vi "Measurement Logic.vi"(8 "error in":errorcluster, 10 "Measurement Context":refnum<class "MeasurementContext.lvclass">, 11 "Measurement Configuration":T2={"pin_name"="Pin1", "measurement_type"=1, "range"=10.0, "resolution_digits"=5.5} {"measurement_type" items=["DC Volts"=1, "AC Volts"=2, "DC Current"=3, "AC Current"=4, "2-Wire Resistance"=5, "4-Wire Resistance"=101, "Frequency"=104, "Period"=105, "AC Volts DC Coupled"=1001, "Diode"=1002, "Waveform Voltage"=1003, "Waveform Current"=1004, "Capacitance"=1005, "Inductance"=1006, "Temperature"=108]}) -> (0 "error out":errorcluster, 2 "Measurement Context out":refnum<class "MeasurementContext.lvclass">, 3 "Measurement Results":T1)   [LabVIEW 2020, in "NI-DMM Measurement.lvlib"]
uses:
  NI-DMM Measurement.lvlib
  Measurement Configuration.ctl
  Measurement Results.ctl
  RPC Service/MeasurementContext/MeasurementContext.lvclass
  measurement-services-labview-DCPowerExample/Source/Session Management Client_lv/MeasurementLink Session Management Client/RPC Messages/ni_measurementlink_sessionmanagement_v1_ReserveSessionsRequest.ctl
  measurement-services-labview-DCPowerExample/Source/Session Management Client_lv/MeasurementLink Session Management Client/RPC Messages/ni_measurementlink_PinMapContext.ctl
  <vilib>/MeasurementLink/Discovery Client/RPC Messages/ni_measurementlink_discovery_v1_ResolveServiceRequest.ctl
  measurement-services-labview-DCPowerExample/Source/Session Management Client_lv/MeasurementLink Session Management Client/MeasurementLink Session Management Client.lvlib
  <vilib>/MeasurementLink/Discovery Client/MeasurementLink Discovery Client.lvlib
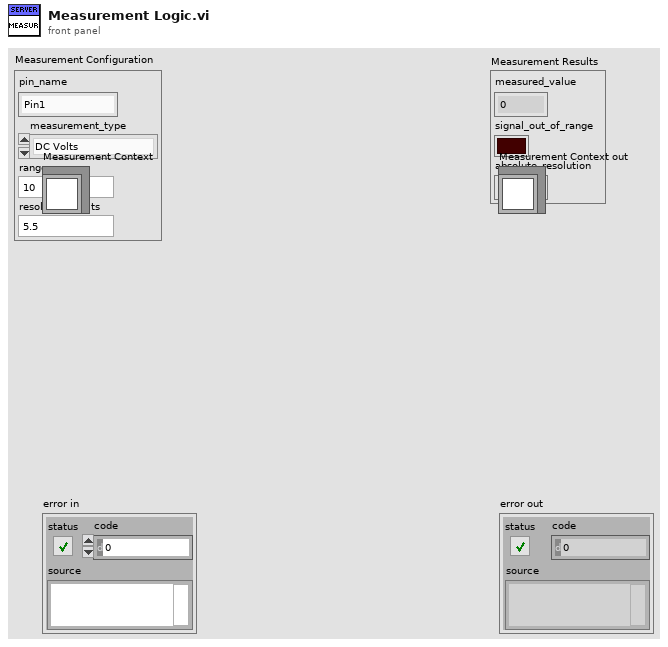
[diagram p1: front panel]
types:
  T1 = typedef "NI-DMM Measurement.lvlib/Measurement Results.ctl" = cluster{"measured_value":dbl, "signal_out_of_range":bool, "absolute_resolution":dbl}
  T2 = typedef "NI-DMM Measurement.lvlib/Measurement Configuration.ctl" = cluster{"pin_name":string, "measurement_type":i32, "range":dbl, "resolution_digits":dbl}
  T3 = typedef "MeasurementLink Discovery Client.lvlib/ni_measurementlink_discovery_v1_ResolveServiceRequest.ctl" = cluster{"provided_interface":string, "service_class":string}
  T4 = typedef "MeasurementLink Session Management Client.lvlib/ni_measurementlink_sessionmanagement_v1_ReserveSessionsRequest.ctl" = cluster{"pin_map_context":T5, "pin_or_relay_names":string[], "instrument_type_id":string, "timeout_in_milliseconds":i32}
  T5 = typedef "MeasurementLink Session Management Client.lvlib/ni_measurementlink_PinMapContext.ctl" = cluster{"pin_map_id":string, "sites":i32[]}
  T6 = typedef "MeasurementLink Measurement Server Internal.lvlib/ni_measurementlink_PinMapContext.ctl" = cluster{"pin_map_id":string, "sites":i32[]}
  T7 = typedef "grpc-lvsupport-release.lvlib/grpcId.ctl" = u64
  T8 = typedef "MeasurementLink Discovery Client.lvlib/ni_measurementlink_discovery_v1_ServiceLocation.ctl" = cluster{"location":string, "insecure_port":string, "ssl_authenticated_port":string}
  T9 = typedef "MeasurementLink Session Management Client.lvlib/ni_measurementlink_sessionmanagement_v1_ReserveSessionsResponse.ctl" = cluster{"sessions":T10[]}
  T10 = typedef "MeasurementLink Session Management Client.lvlib/ni_measurementlink_sessionmanagement_v1_SessionInformation.ctl" = cluster{"session":T11, "resource_name":string, "channel_list":string, "instrument_type_id":string, "session_exists":bool}
  T11 = typedef "MeasurementLink Session Management Client.lvlib/ni_measurementlink_sessionmanagement_v1_Session.ctl" = cluster{"name":string}
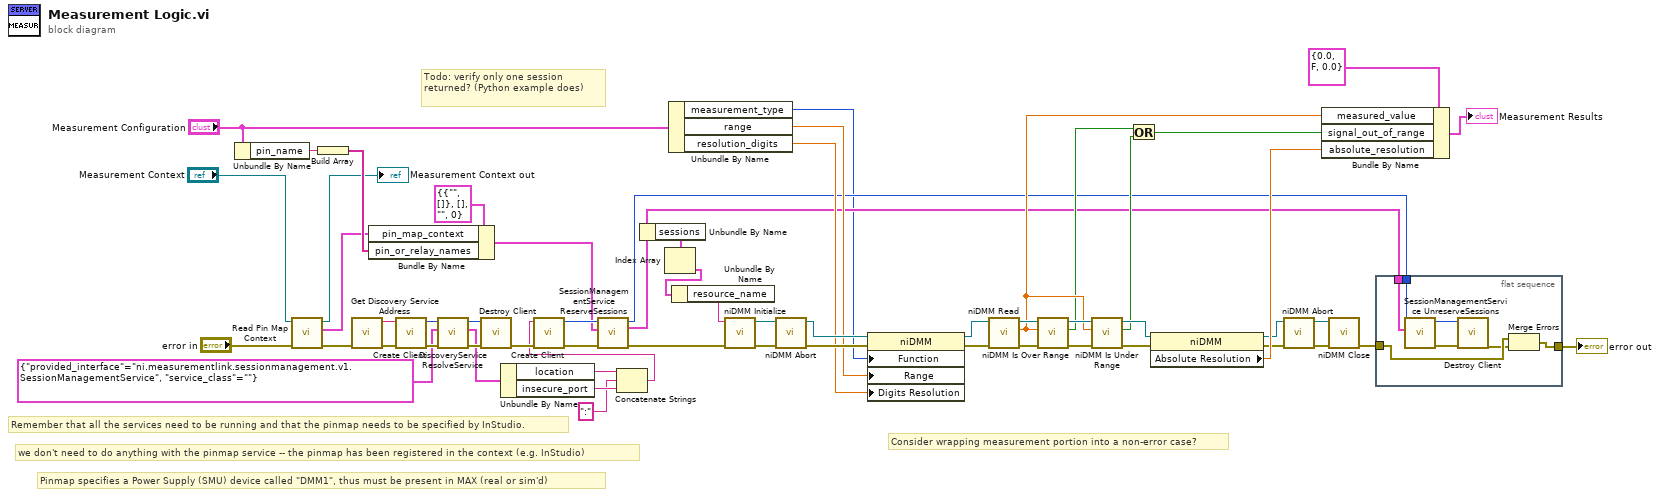
[diagram p0: block diagram]
diagram:
  # "Consider wrapping measurement portion into a non-error case?"
  # "Todo: verify only one session returned? (Python example does)"
  # "Pinmap specifies a Power Supply (SMU) device called \"DMM1\", thus must be present in MAX (real or sim'd)"
  # "Remember that all the services need to be running and that the pinmap needs to be specified by InStudio."
  # "we don't need to do anything with the pinmap service -- the pinmap has been registered in the context (e.g. InStudio)"
  n1 = Unbundle By Name("Measurement Configuration") -> ("pin_name"=w59:string)
  n2 = call-dynamic "Read Pin Map Context.vi"("error in (no error)"="error in", "MeasurementContext in"="Measurement Context") -> ("error out"=w37:errorcluster, "pin map context"=w54:T6, "MeasurementContext out"=→"Measurement Context out":refnum<class "MeasurementContext.lvclass">)  [unwired: 7 in]
  n3 = Build Array(w59) -> (w58:string[])
  n4 = call "Get Discovery Service Address.vi"("error in"=w37) -> ("error out"=w36:errorcluster, "address"=w35:string)  [unwired: 9 in]
  n5 = Bundle By Name(cluster=T4 {"pin_map_context"={"pin_map_id"="", "sites"=[]}, "pin_or_relay_names"=[], "instrument_type_id"="", "timeout_in_milliseconds"=0} ("Request Data"), "pin_map_context"=w54, "pin_or_relay_names"=w58) -> (w50:T4)
  n6 = call <vilib>:"Create Client.vi"("error in"=w36, "address"=w35) -> ("error out"=w47:errorcluster, "gRPC ID Out"=w46:T7)  [unwired: 8 in]
  n7 = call <vilib>:"DiscoveryService ResolveService.vi"("error in"=w47, "Request Data"=T3 {"provided_interface"="ni.measurementlink.sessionmanagement.v1.SessionManagementService", "service_class"=""}, "gRPC ID"=w46) -> ("error out"=w44:errorcluster, "Response Data"=w39:T8, "gRPC ID out"=w45:T7)  [unwired: 6 in]
  n8 = call <vilib>:"Destroy Client.vi"("error in"=w44, "gRPC ID"=w45) -> ("error out"=w43:errorcluster)  [unwired: 9 in]
  n9 = Unbundle By Name(w39) -> ("location"=w42:string, "insecure_port"=w41:string)
  n10 = Concatenate Strings(w42, ":" ("string"), w41) -> (w38:string)
  n11 = call <vilib>:"Create Client.vi"("error in"=w43, "address"=w38) -> ("error out"=w56:errorcluster, "gRPC ID Out"=w57:T7)  [unwired: 8 in]
  n12 = call "SessionManagementService ReserveSessions.vi"("error in"=w56, "Request Data"=w50, "gRPC ID"=w57) -> ("error out"=w31:errorcluster, "Response Data"=w4:T9, "gRPC ID out"=w7:T7)  [unwired: 6 in]
  n13 = Unbundle By Name(w4) -> ("sessions"=w49:T10[])
  n14 = Index Array(array=w49) -> (element=w48:T10)  [unwired: 1 in]
  n15 = Unbundle By Name("Measurement Configuration") -> ("measurement_type"=w3:i32, "range"=w24:dbl, "resolution_digits"=w23:dbl)
  n16 = Unbundle By Name(w48) -> ("resource_name"=w30:string)
  n17 = call <instrlib>:"niDMM Initialize.vi"("error in (no error)"=w31, "Instrument Descriptor"=w30) -> ("error out"=w27:errorcluster, "instrument handle out"=w26:refnum<k15>)  [unwired: 8 in]
  n18 = call <instrlib>:"niDMM Abort.vi"("error in (no error)"=w27, "instrument handle"=w26) -> ("error out"=w29:errorcluster, "instrument handle out"=w28:refnum<k15>)  [unwired: 8 in]
  n19 = property class="niDMM"(reference=w28, error in=w29, "Function"=w3, "Range"=w24, "Digits Resolution"=w23) -> (reference out=w21:refnum<k15>, error out=w22:errorcluster)
  n20 = call <instrlib>:"niDMM Read.vi"("error in (no error)"=w22, "instrument handle"=w21) -> ("error out"=w17:errorcluster, "Measurement"=w13:dbl, "instrument handle out"=w16:refnum<k15>)  [unwired: 7 in]
  n21 = call <instrlib>:"niDMM Is Over Range.vi"("error in (no error)"=w17, "Measurement"=w13, "instrument handle"=w16) -> ("error out"=w12:errorcluster, "Over Range?"=w10:bool, "instrument handle out"=w14:refnum<k15>)  [unwired: 6 in]
  n22 = call <instrlib>:"niDMM Is Under Range.vi"("error in (no error)"=w12, "Measurement"=w13, "instrument handle"=w14) -> ("error out"=w11:errorcluster, "Under Range?"=w8:bool, "instrument handle out"=w15:refnum<k15>)  [unwired: 6 in]
  n23 = Or(x=w10, y=w8) -> (x .or. y?=w9:bool)
  n24 = property class="niDMM"(reference=w15, error in=w11) -> (reference out=w18:refnum<k15>, error out=w19:errorcluster, "Absolute Resolution"=w20:dbl)
  n25 = call <instrlib>:"niDMM Abort.vi"("error in (no error)"=w19, "instrument handle"=w18) -> ("error out"=w6:errorcluster, "instrument handle out"=w5:refnum<k15>)  [unwired: 8 in]
  n26 = Bundle By Name(cluster=T1 {"measured_value"=0.0, "signal_out_of_range"=FALSE, "absolute_resolution"=0.0} ("Measurement Results"), "measured_value"=w13, "signal_out_of_range"=w9, "absolute_resolution"=w20) -> (→"Measurement Results":T1)
  n27 = call <instrlib>:"niDMM Close.vi"("error in (no error)"=w6, "instrument handle"=w5) -> ("error out"=w2:errorcluster)  [unwired: 9 in]
  n28 = flat-sequence {
    tunnel: w7 -> [w64]
    tunnel: w4 -> [w63]
    tunnel: w2 -> [w62]
    tunnel: [w60] -> w1
    frame #0 {
      n29 = call "SessionManagementService UnreserveSessions.vi"("Request Data"=w63, "gRPC ID"=w64) -> ("error out"=w65:errorcluster, "gRPC ID out"=w66:T7)  [unwired: 7 in, 1 out]
      n30 = call <vilib>:"Destroy Client.vi"("error in"=w65, "gRPC ID"=w66) -> ("error out"=w61:errorcluster)  [unwired: 9 in]
      n31 = Merge Errors(w62, w61) -> (w60:errorcluster)
    }
  }
  "error out" <- w1
